vi "testing_node.vi"() -> ()   [LabVIEW 2018]
uses:
  <vilib>/Utility/xml.llb/Read From XML File(string).vi
panel:
  out "Success Rate":dbl
  in  "Test Data Folder":path
  in  "Weights XML\n(Select Existing File)":path
  in  "Expected Output":dbl[](array[numeric])
  out "Output":dbl[](array[numeric])
  # "Neural Network Testing Node"
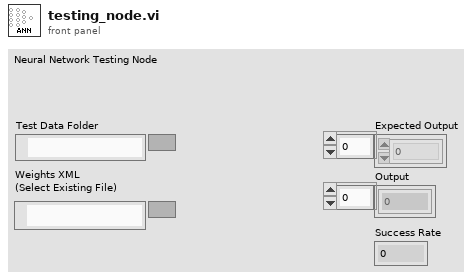
[diagram p1: front panel]
types:
  T1 = cluster{cluster{dbl[][], dbl[][], dbl[][]}, cluster{dbl[], dbl[], dbl[]}}
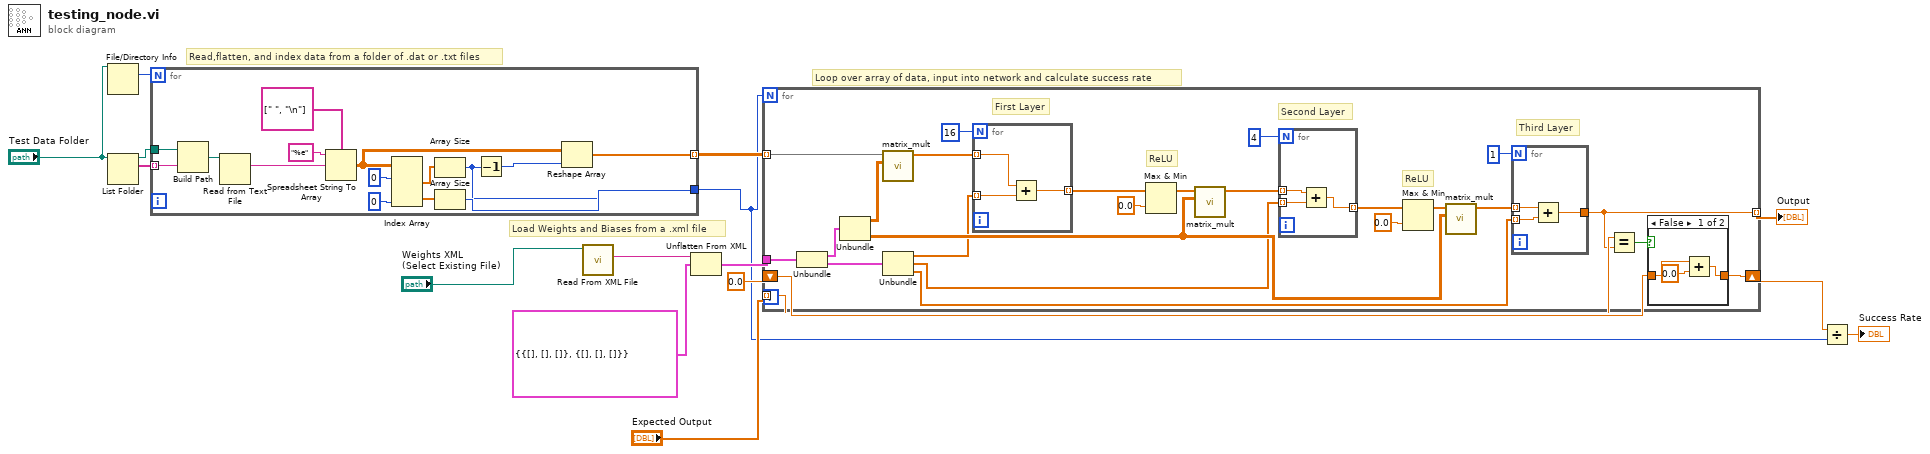
[diagram p0: block diagram]
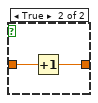
[diagram p2: hidden frame]
diagram:
  # "Load Weights and Biases from a .xml file"
  # "Loop over array of data, input into network and calculate success rate"
  # "Read,flatten, and index data from a folder of .dat or .txt files"
  n1 = File/Directory Info(path="Test Data Folder") -> (size=w10:i64)  [unwired: 1 in, 6 out]
  n2 = List Folder(path="Test Data Folder") -> (path out=w12:path, filenames=w13:string[])  [unwired: 3 in, 2 out]
  n3 = for {
    N: w10 -> [_]
    tunnel: w13 -> [w30] mode=indexing
    tunnel: w12 -> [w29]
    tunnel: [w20] -> w2
    tunnel: [w17] -> _
    tunnel: [w16] -> w9 mode=indexing
    n4 = Build Path(base path=w29, name or relative path=w30) -> (appended path=w28:path)
    n5 = Read from Text File(file (use dialog)=w28) -> (text=w26:string)  [unwired: 3 in, 3 out]
    n6 = Spreadsheet String To Array(delimiter (Tab)=string[] [" ", "\n"], format string="%e", spreadsheet string=w26) -> (array=w19:dbl[][])  [unwired: 1 in]
    n7 = Index Array(array=w19, index (row) #1=0 ("index (row)"), index (col) #2=0 ("disabled index (col)")) -> (element #1=w23:dbl[], element #2=w21:dbl[])  [unwired: 2 in]
    n8 = Array Size(array=w23) -> (size(s)=w17:i32)
    n9 = Array Size(array=w21) -> (size(s)=w20:i32)
    n10 = Decrement(x=w17) -> (x-1=w18:i32)
    n11 = Reshape Array(w19, w18) -> (w16:dbl[])
  }
  n12 = call-poly <vilib>:"Read From XML File.vi"("XML File Path"="Weights XML\n(Select Existing File)") -> ("XML Elements"=w6:string)  [unwired: 8 in, 2 out]
  n13 = Unflatten From XML(xml string=w6, type=T1 {{[], [], []}, {[], [], []}}) -> (value=w7:T1)  [unwired: 1 in, 1 out]
  n14 = for {
    N: w2 -> [_]
    tunnel: "Expected Output" -> [w35] mode=indexing
    tunnel: w9 -> [w37] mode=indexing
    tunnel: [w34] -> w8 mode=indexing
    tunnel: w7 -> [w43]
    shift-right: [w31] -> w3
    shift-left: 0.0 -> [w32]
    # "Third Layer"
    # "Second Layer"
    # "First Layer"
    # "ReLU"
    # "ReLU"
    n15 = Unbundle(w43) -> (w39:cluster{dbl[][], dbl[][], dbl[][]}, w38:cluster{dbl[], dbl[], dbl[]})
    n16 = Unbundle(w39) -> (w48:dbl[][], w47:dbl[][])  [unwired: 1 out]
    n17 = call "matrix_mult.vi"("Weights"=w48, "Input Array"=w37) -> ("Matrix Product"=w36:dbl[])  [unwired: 9 in]
    n18 = Unbundle(w38) -> (w46:dbl[], w45:dbl[], w44:dbl[])
    n19 = for {
      N: 16 -> [_]
      tunnel: [w70] -> w56 mode=indexing
      tunnel: w36 -> [w69] mode=indexing
      tunnel: w46 -> [w68] mode=indexing
      n20 = Add(x=w69, y=w68) -> (x+y=w70:dbl)
    }
    n21 = Max & Min(x=w56, y=0.0) -> (max(x,y)=w42:dbl[])  [unwired: 1 out]
    n22 = call "matrix_mult.vi"("Weights"=w47, "Input Array"=w42) -> ("Matrix Product"=w41:dbl[])  [unwired: 9 in]
    n23 = for {
      N: 4 -> [_]
      tunnel: [w67] -> w50 mode=indexing
      tunnel: w41 -> [w66] mode=indexing
      tunnel: w45 -> [w65] mode=indexing
      n24 = Add(x=w66, y=w65) -> (x+y=w67:dbl)
    }
    n25 = Max & Min(x=w50, y=0.0) -> (max(x,y)=w40:dbl[])  [unwired: 1 out]
    n26 = call "matrix_mult.vi"("Weights"=w47, "Input Array"=w40) -> ("Matrix Product"=w49:dbl[])  [unwired: 9 in]
    n27 = for {
      N: 1 -> [_]
      tunnel: [w64] -> w34
      tunnel: w49 -> [w63] mode=indexing
      tunnel: w44 -> [w62] mode=indexing
      n28 = Add(x=w63, y=w62) -> (x+y=w64:dbl)
    }
    n29 = Equal?(x=w35, y=w34) -> (x = y?=w33:bool)
    n30 = case shown="False" w33 {
      tunnel: w32 -> [w59 w61]
      tunnel: [w57 w60] -> w31
      frame False {
        n31 = Add(x=w59, y=0.0) -> (x+y=w57:dbl)
      }
      frame True {
        n32 = Increment(x=w61) -> (x+1=w60:dbl)
      }
    }
  }
  "Output" <- w8
  n33 = Divide(x=w3, y=w2) -> (x/y=→"Success Rate":dbl)
